vi "get_drive_status.vi"(8 "error in (no error)":errorcluster, 10 "Device ID":i32, 11 "Handle in":i64) -> (0 "error out":errorcluster, 2 "Return (<0 is error)":i32, 3 "Handle out":i64)   [LabVIEW 2016, in "OSB_uMp_library.lvlib"]
doc: "Returns 0 if uMp is idle.\n\n!!!\nUsage warning\n!!!\nMay need to get recent information from the uMp before calling this VI. One way of doing this is to call the \"ping\" VI first."
uses:
  OSB_uMp_library.lvlib
  ump.dll
panel:
  # "By Stuart Box at OxSyBio Ltd, 2017\n\nThis software is provided WITHOUT ANY WARRANTY; without even the implied warranty of MERCHANTABILITY or FITNESS FOR A PARTICULAR PURPOSE.\n\ninfo@oxsybio.com\n\nOxSyBio Ltd, The Walbrook Building, 25 Walbrook, London, EC4N 8AF"
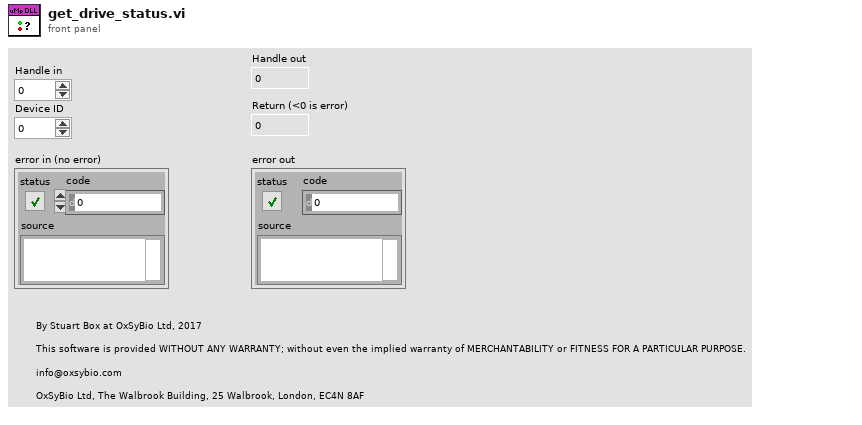
[diagram p1: front panel]
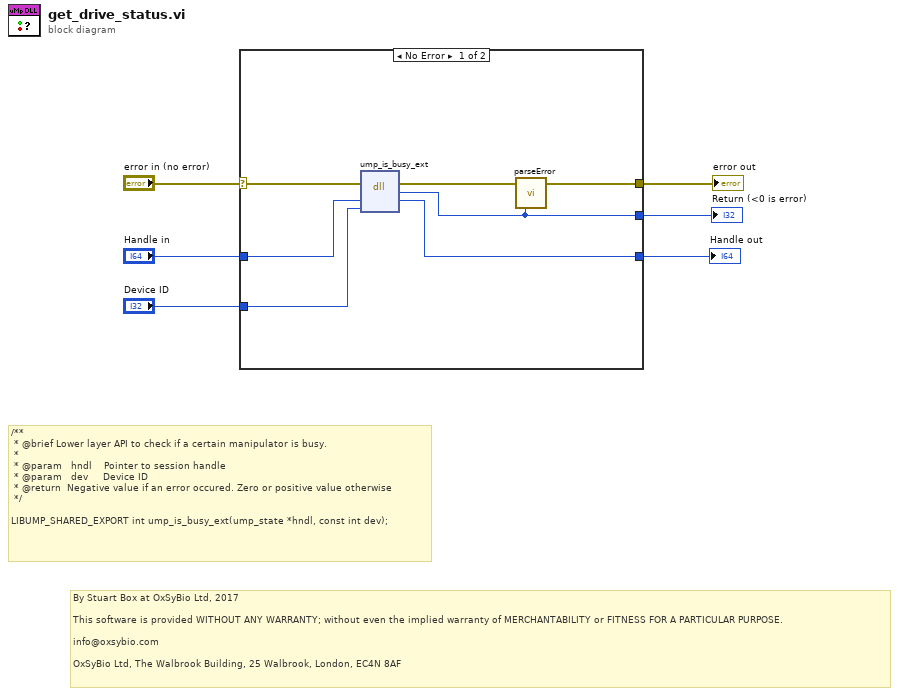
[diagram p0: block diagram]
diagram:
  # "By Stuart Box at OxSyBio Ltd, 2017\n\nThis software is provided WITHOUT ANY WARRANTY; without even the implied warranty of MERCHANTABILITY or FITNESS FOR A PARTICULAR PURPOSE.\n\ninfo@oxsybio.com\n\nOxSyBio Ltd, The Walbrook Building, 25 Walbrook, London, EC4N 8AF"
  # "/**\n * @brief Lower layer API to check if a certain manipulator is busy.\n *\n * @param   hndl    Pointer to session handle\n * @param   dev     Device ID\n * @return  Negative value if an error occured. Zero or positive value otherwise\n */\n\nLIBUMP_SHARED_EXPORT int ump_is_busy_ext(ump_state *hndl, const int dev);"
  n1 = case shown="No Error" "error in (no error)" {
    selector: "error in (no error)" -> [w12 w15]
    tunnel: [w7 _] -> w6
    tunnel: [w8 w15] -> w5
    tunnel: "Handle in" -> [w13 w14]
    tunnel: [w11 w14] -> w2
    tunnel: "Device ID" -> [w10 _]
    frame No Error {
      n2 = dll-call lib="C:/Users/Stu/Desktop/OSB LabVIEW uMp/uMp_library/ump.dll" fn="ump_is_busy_ext"(error in=w12, "handle"=w13, "dev"=w10) -> (error out=w9:errorcluster, "return"=w7:i32, "handle"=w11:i64)  [unwired: 3 in, 1 out]
      n3 = call "parseError.vi"("Error In"=w9, "ump dll return value (<0 is error)"=w7) -> ("Error Out"=w8:errorcluster)  [unwired: 24 in, 1 out]
    }
    frame Error {
    }
  }
  "Return (<0 is error)" <- w6
  "error out" <- w5
  "Handle out" <- w2
